vi "ble_dongle_info.vi"(8 "error in (no error)":errorcluster, 11 "COM Bluegiga in":refnum<visa-resource-name>) -> (0 "error out":errorcluster, 2 "info":string, 3 "COM Bluegiga out":refnum<visa-resource-name>)   [LabVIEW 2013]
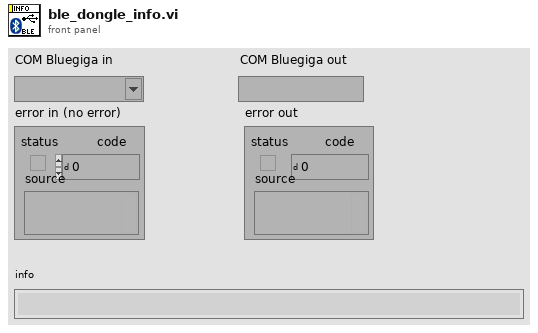
[diagram p1: front panel]
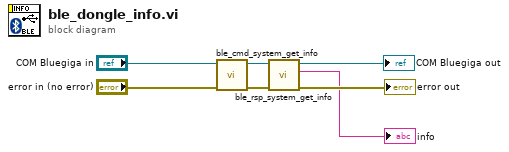
[diagram p0: block diagram]
diagram:
  n1 = call "ble_cmd_system_get_info.vi"("error in (no error)"="error in (no error)", "COM Bluegiga in"="COM Bluegiga in") -> ("error out"=w5:errorcluster, "COM Bluegiga out"=w4:refnum<visa-resource-name>)  [unwired: 8 in]
  n2 = call "ble_rsp_system_get_info.vi"("error in (no error)"=w5, "COM Bluegiga in"=w4) -> ("error out"=→"error out":errorcluster, "info"=→"info":string, "COM Bluegiga out"=→"COM Bluegiga out":refnum<visa-resource-name>)  [unwired: 6 in, 1 out]
